vi "Open VIs.vi"(8 "error in (no error)":errorcluster, 9 "Title Prefix In":string, 10 "VI Screenshots":T1, 11 "VI Path":path) -> (0 "error out":errorcluster, 2 "VI Screenshots out":T1)   [LabVIEW 2015, in "VIDiff_Utilities.lvlib"]
uses:
  VIDiff_Utilities.lvlib
  Screenshots/VI Screenshots.ctl
  Screenshots/Screenshot Info.ctl
  Screenshots/Screenshot Type.ctl
  FilePaths.ctl
  Screenshots/VIDiff_Screenshots.lvlib
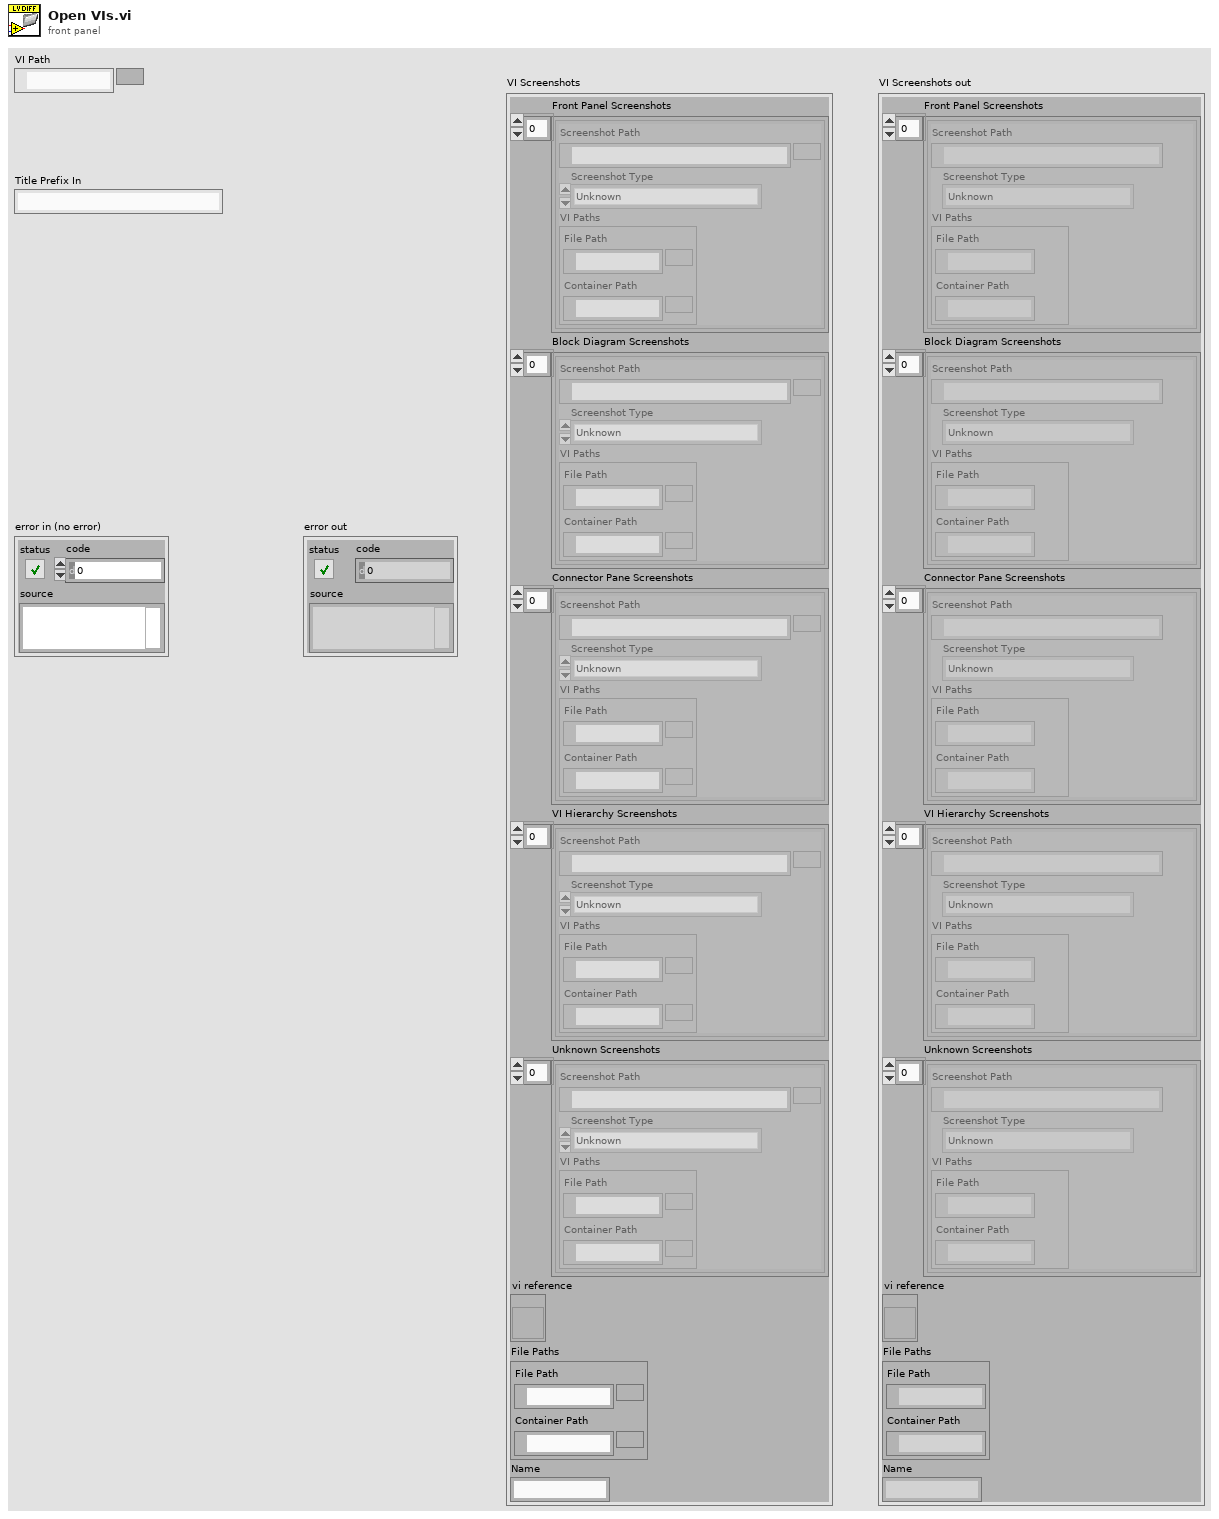
[diagram p1: front panel]
types:
  T1 = typedef "VIDiff_Screenshots.lvlib/VI Screenshots.ctl" = cluster{"Front Panel Screenshots":T2[], "Block Diagram Screenshots":T2[], "Connector Pane Screenshots":T2[], "VI Hierarchy Screenshots":T2[], "Unknown Screenshots":T2[], "vi reference":refnum<vi>, "File Paths":cluster{"File Path":path, "Container Path":path}, "Name":string}
  T2 = typedef "VIDiff_Screenshots.lvlib/Screenshot Info.ctl" = cluster{"Screenshot Path":path, "Screenshot Type":T3, "VI Paths":T4}
  T3 = typedef "VIDiff_Screenshots.lvlib/Screenshot Type.ctl" = enum16{"Unknown", "Front Panel", "Connector Pane", "Block Diagram", "VI Hierarchy"}
  T4 = typedef "VIDiff_Utilities.lvlib/FilePaths.ctl" = cluster{"File Path":path, "Container Path":path}
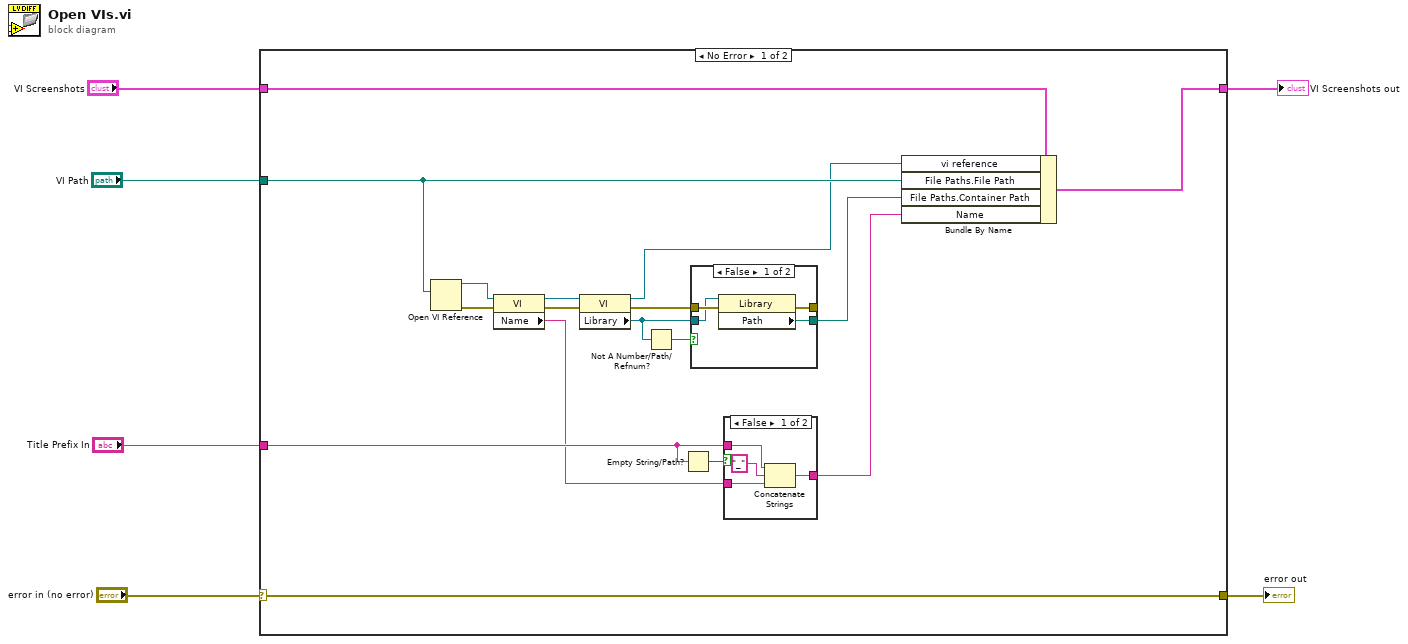
[diagram p0: block diagram]
diagram:
  n1 = case shown="No Error" "error in (no error)" {
    selector: "error in (no error)" -> [w22 w35]
    tunnel: [w22 w35] -> w5
    tunnel: "VI Screenshots" -> [w19 w34]
    tunnel: [w17 w34] -> w3
    tunnel: "VI Path" -> [w16 _]
    tunnel: "Title Prefix In" -> [w9 _]
    frame No Error {
      n2 = Open VI Reference(vi path=w16) -> (vi reference=w15:refnum<vi>, error out=w14:errorcluster)  [unwired: 5 in]
      n3 = property class="VI"(reference=w15, error in=w14) -> (reference out=w12:refnum<vi>, error out=w13:errorcluster, "Name"=w8:string)
      n4 = property class="VI"(reference=w12, error in=w13) -> (reference out=w11:refnum<vi>, error out=w23:errorcluster, "Library"=w20:refnum<vi>)
      n5 = Not A Number/Path/Refnum?(number/path/refnum=w20) -> (NaN/Path/Refnum?=w21:bool)
      n6 = Empty String/Path?(string/path=w9) -> (empty?=w10:bool)
      n7 = case shown="False" w21 {
        tunnel: [w32 _] -> w18
        tunnel: w23 -> [w31 w33]
        tunnel: [w30 w33] -> _
        tunnel: w20 -> [w29 _]
        frame False {
          n8 = property class="Library"(reference=w29, error in=w31) -> (error out=w30:errorcluster, "Path"=w32:path)  [unwired: 1 out]
        }
        frame True {
        }
      }
      n9 = case shown="False" w10 {
        tunnel: w8 -> [w27 w28]
        tunnel: [w26 w28] -> w7
        tunnel: w9 -> [w24 _]
        frame False {
          n10 = Concatenate Strings(w24, "_" ("string"), w27) -> (w26:string)
        }
        frame True {
        }
      }
      n11 = Bundle By Name(cluster=w19, "vi reference"=w11, "File Paths.File Path"=w16, "File Paths.Container Path"=w18, "Name"=w7) -> (w17:T1)
    }
    frame Error {
    }
  }
  "error out" <- w5
  "VI Screenshots out" <- w3
